vi "ping.vi"(8 "error in (no error)":errorcluster, 9 "timeout (ms)":i32=100, 10 "SetSize":i32=32, 11 "IP/Address":string="127.0.0.1") -> (0 "error out":errorcluster, 1 "RoundtripTime":i64, 2 "Status":i32(ring) items=["Success"=0, "DestinationNetworkUnreachable"=11002, "DestinationHostUnreachable"=11003, "DestinationProhibited, DestinationProtocolUnreachable"=11004, "DestinationPortUnreachable"=11005, "NoResources"=11006, "BadOption"=11007, "HardwareError"=11008, "PacketTooBig"=11009, "TimedOut"=11010, "BadRoute"=11012, "TtlExpired"=11013, "TtlReassemblyTimeExceeded"=11014, "ParameterProblem"=11015, "SourceQuench"=11016, "BadDestination"=11018, "DestinationUnreachable"=11040, "TimeExceeded"=11041, "BadHeader"=11042, "UnrecognizedNextHeader"=11043, "IcmpError"=11044, "DestinationScopeMismatch"=11045, "Unknown"=-1], 3 "Success?":bool)   [LabVIEW 2026, in "TALOS.lvlib"]
uses:
  TALOS.lvlib
  Ancestor/Ancestor/Ancestor.lvclass/Ancestor.ctl
  Generate Error.vi
  FGV/Error Memory/Get Error Description.vi
  Get PC name.vi
  Ancestor/Ancestor/Read ID.vi
  Get Class Name.vi
  <vilib>/Utility/error.llb/Clear Errors.vi
  FGV/Error Memory/Error Memory Core.vi
  <vilib>/AdvancedString/Delimited String to 1D String Array.vi
  <vilib>/AdvancedString/Delimited String to 1D String Array (string).vi
  Circus Root Path.vi
  FGV/Error Memory/Error Crt Lvl checker.vi
  FGV/Error Memory/Error Memory Core.vi/40c8088d-b597-4017-91af-faa98e00292e.vi
  FGV/Error Memory/Error Memory Core.vi/d4a3ab98-063c-4e44-b43d-fbdcfe6c2be2.vi
  Global Memory.vi
  <vilib>/Utility/LVClass/Get LV Class Name.vi
  Is in Packed Library.vi
  TALOS Root path.vi
  Read CSV worksheet.vi
  Global Constants.vi
  <vilib>/Utility/error.llb/General Error Handler.vi
  Error Log.vi
  Ancestor/Ancestor/Ancestor.lvclass
  <vilib>/Comparison/Equal/Equal Functor/Equal Functor.lvclass
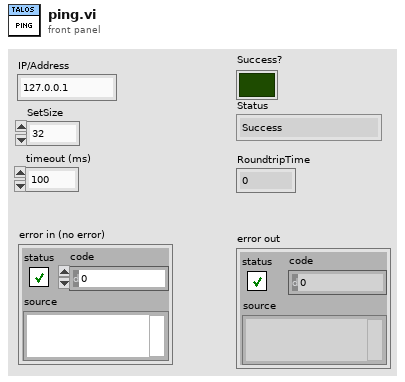
[diagram p1: front panel]
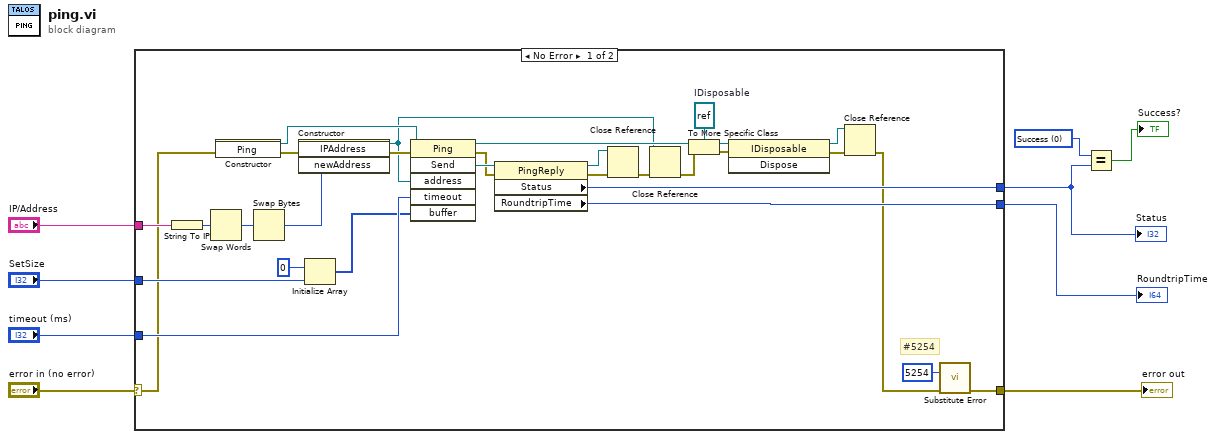
[diagram p0: block diagram]
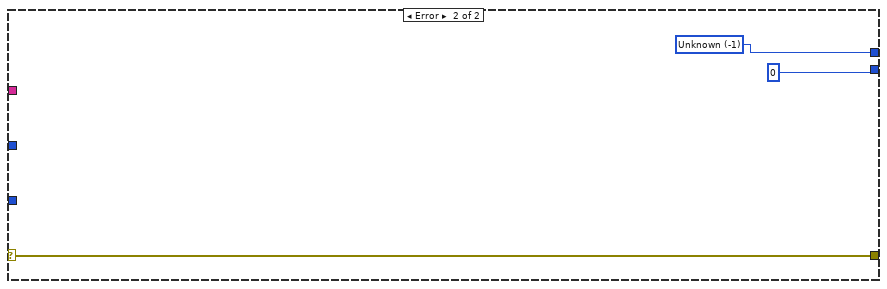
[diagram p2: hidden frame]
diagram:
  w3 = 0 items=["Success"=0, "DestinationNetworkUnreachable"=11002, "DestinationHostUnreachable"=11003, "DestinationProhibited, DestinationProtocolUnreachable"=11004, "DestinationPortUnreachable"=11005, "NoResources"=11006, "BadOption"=11007, "HardwareError"=11008, "PacketTooBig"=11009, "TimedOut"=11010, "BadRoute"=11012, "TtlExpired"=11013, "TtlReassemblyTimeExceeded"=11014, "ParameterProblem"=11015, "SourceQuench"=11016, "BadDestination"=11018, "DestinationUnreachable"=11040, "TimeExceeded"=11041, "BadHeader"=11042, "UnrecognizedNextHeader"=11043, "IcmpError"=11044, "DestinationScopeMismatch"=11045, "Unknown"=-1] ("Status")
  n1 = case shown="No Error" "error in (no error)" {
    selector: "error in (no error)" -> [w34 w42]
    tunnel: "IP/Address" -> [w39 _]
    tunnel: "timeout (ms)" -> [w38 _]
    tunnel: "SetSize" -> [w37 _]
    tunnel: [w36 w40] -> w2
    tunnel: [w35 i64 0 ("RoundtripTime")] -> w6
    tunnel: [w10 w42] -> w4
    frame No Error {
      w22 = refnum<k24> refnum  # IDisposable
      # "#5254"
      n2 = String To IP(1:w39) -> (0:w26:u32)
      n3 = Swap Words(1:w26) -> (0:w24:u32)
      n4 = constructor class="Ping"(error in=w34) -> (reference out=w31:refnum<k24>, error out=w28:errorcluster)  [unwired: 2 in, 1 out]
      n5 = Swap Bytes(anything=w24) -> (byte swapped=w25:u32)
      n6 = constructor class="IPAddress"(error in=w28, "newAddress"=w25) -> (reference out=w18:refnum<k24>, error out=w27:errorcluster)  [unwired: 2 in, 2 out]
      n7 = Initialize Array(u8 0, w37) -> (w30:u8[])
      n8 = invoke class="Ping" method="Send"(reference=w31, error in=w27, "address"=w18, "timeout"=w38, "buffer"=w30) -> (reference out=w23:refnum<k24>, error out=w32:errorcluster, "Send"=w33:refnum<k24>)  [unwired: 1 in, 3 out]
      n9 = property class="PingReply"(reference=w33, error in=w32) -> (reference out=w21:refnum<k24>, error out=w20:errorcluster, "Status"=w36:i32, "RoundtripTime"=w35:i64)
      n10 = Close Reference(reference=w21, error in (no error)=w20) -> (error out=w19:errorcluster)
      n11 = Close Reference(reference=w18, error in (no error)=w19) -> (error out=w17:errorcluster)
      n12 = To More Specific Class(target class=w22, reference=w23, error in=w17) -> (specific class reference=w16:refnum<k24>, error out=w15:errorcluster)
      n13 = invoke class="IDisposable" method="Dispose"(reference=w16, error in=w15) -> (reference out=w13:refnum<k24>, error out=w14:errorcluster)  [unwired: 1 in, 1 out]
      n14 = Close Reference(reference=w13, error in (no error)=w14) -> (error out=w11:errorcluster)
      n15 = call "Substitute Error.vi"("error in (no error)"=w11, "Error Code"=5254) -> ("error out"=w10:errorcluster)  [unwired: 9 in]
    }
    frame Error {
      w40 = -1 items=["Success"=0, "DestinationNetworkUnreachable"=11002, "DestinationHostUnreachable"=11003, "DestinationProhibited, DestinationProtocolUnreachable"=11004, "DestinationPortUnreachable"=11005, "NoResources"=11006, "BadOption"=11007, "HardwareError"=11008, "PacketTooBig"=11009, "TimedOut"=11010, "BadRoute"=11012, "TtlExpired"=11013, "TtlReassemblyTimeExceeded"=11014, "ParameterProblem"=11015, "SourceQuench"=11016, "BadDestination"=11018, "DestinationUnreachable"=11040, "TimeExceeded"=11041, "BadHeader"=11042, "UnrecognizedNextHeader"=11043, "IcmpError"=11044, "DestinationScopeMismatch"=11045, "Unknown"=-1] ("Status")
    }
  }
  "RoundtripTime" <- w6
  "error out" <- w4
  "Status" <- w2
  n16 = Equal?(x=w3, y=w2) -> (x = y?=→"Success?":bool)
